vi "_builtins_arrange_panel.vi"(8 "error in (no error)":errorcluster, 10 "Arrange":T1, 11 "VI Refnum in":refnum<vi>) -> (0 "error out":errorcluster, 3 "VI Refnum out":refnum<vi>)   [LabVIEW 2019, in "Script.lvlib"]
doc: "Arranges the selected controls to the panel grid by left or top edges (hold shift). If nothing is selected, this will arrange all the controls on the panel into columns with a dead zone offset from the panel origin.\n\nCreated by: Ryan Pacini"
uses:
  Script.lvlib
  _builtins_arrange.ctl
  _builtins_align.ctl
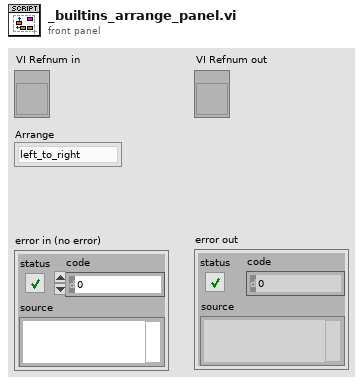
[diagram p1: front panel]
types:
  T1 = typedef "Script.lvlib/_builtins_arrange.ctl" = enum8{"left_to_right", "right_to_left"}
  T2 = typedef "Script.lvlib/_builtins_align.ctl" = enum8{"Top Edges", "Vertical Centers", "Bottom Edges", "Left Edges", "Horizontal Centers", "Right Edges"}
  T3 = typedef "LVRectTypeDef.ctl" = cluster{"Left":i16, "Top":i16, "Right":i16, "Bottom":i16}
  T4 = typedef "LVPositionTypeDef.ctl" = cluster{"Left":i32, "Top":i32}
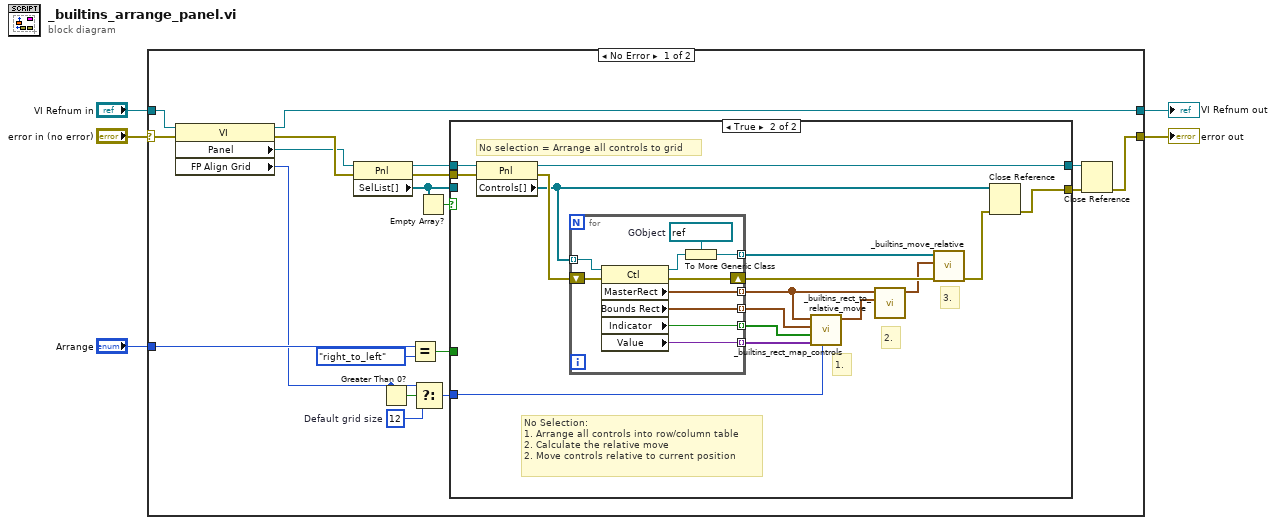
[diagram p0: block diagram]
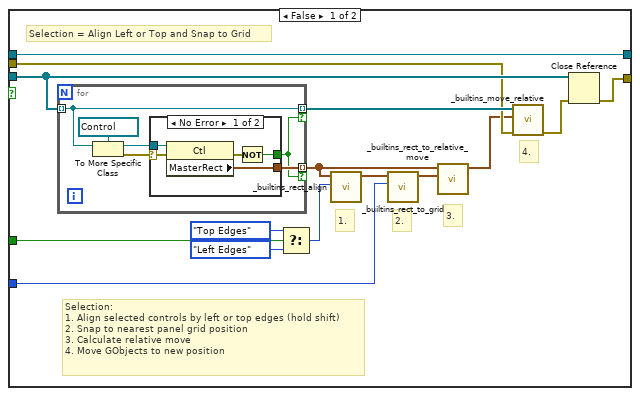
[diagram p2: hidden frame]
diagram:
  n1 = case shown="No Error" "error in (no error)" {
    selector: "error in (no error)" -> [w23 w77]
    tunnel: "VI Refnum in" -> [w24 w78]
    tunnel: [w18 w78] -> w4
    tunnel: [w19 w77] -> w2
    tunnel: "Arrange" -> [w11 _]
    frame No Error {
      w8 = 12  # Default grid size
      n2 = property class="VI"(reference=w24, error in=w23) -> (reference out=w18:refnum<vi>, error out=w22:errorcluster, "Panel"=w21:refnum<vi>, "FP Align Grid"=w7:i32)
      n3 = property class="Pnl"(reference=w21, error in=w22) -> (reference out=w13:refnum<vi>, error out=w16:errorcluster, "SelList[]"=w17:refnum<vi>[])
      n4 = Greater Than 0?(x=w7) -> (x > 0?=w9:bool)
      n5 = Equal?(x=w11, y=_builtins_arrange."right_to_left") -> (x = y?=w10:bool)
      n6 = Select(t=w7, s=w9, f=w8) -> (s? t:f=w6:i32)
      n7 = Empty Array?(array=w17) -> (empty?=w15:bool)
      n8 = case shown="True" w15 {
        tunnel: [w39 w58] -> w20
        tunnel: w17 -> [w36 _]
        tunnel: w16 -> [w32 w64]
        tunnel: [w31 w65] -> w14
        tunnel: w13 -> [w31 w66]
        tunnel: w6 -> [w28 w55]
        tunnel: w10 -> [w29 _]
        frame False {
          # "3."
          # "Selection:\n1. Align selected controls by left or top edges (hold shift)\n2. Snap to nearest panel grid position\n3. Calculate relative move\n4. Move GObjects to new position"
          # "2."
          # "4."
          # "1."
          # "Selection = Align Left or Top and Snap to Grid"
          n9 = for {
            tunnel: w36 -> [w40] mode=indexing
            tunnel: [w40] -> w38 mode=indexing if=w41
            tunnel: [w44] -> w27 mode=indexing if=w41
            n10 = To More Specific Class(target class=refnum<vi> refnum, reference=w40) -> (specific class reference=w42:refnum<vi>, error out=w43:errorcluster)  [unwired: 1 in]
            n11 = case shown="No Error" w43 {
              selector: w43 -> [w49 _]
              tunnel: [w50 _] -> w44
              tunnel: w42 -> [w48 _]
              tunnel: [w47 _] -> w41
              frame No Error {
                n12 = property class="Ctl"(reference=w48, error in=w49) -> (error out=w46:errorcluster, "MasterRect"=w50:T3)  [unwired: 1 out]
                n13 = Not(x=w46) -> (.not. x?=w47:bool)
              }
              frame Error {
              }
            }
          }
          n14 = Select(t=_builtins_align."Top Edges" ("Align Type"), s=w29, f=_builtins_align."Left Edges" ("Align Type")) -> (s? t:f=w33:T2)
          n15 = call "_builtins_rect_align.vi"("Align Type"=w33, "Rects in"=w27) -> ("Resolved Rects out"=w30:T3[])  [unwired: 9 in]
          n16 = call "_builtins_rect_to_grid.vi"("Grid Size (12px)"=w28, "Rects in"=w30) -> ("Resolved Rects out"=w26:T3[])  [unwired: 9 in]
          n17 = call "_builtins_rect_to_relative_move.vi"("End Rects out"=w26, "Start Rects in"=w27) -> ("Relative Move"=w25:T4[])  [unwired: 9 in]
          n18 = call "_builtins_move_relative.vi"("error in (no error)"=w32, "Relative Moves in"=w25, "GObjects in"=w38) -> ("error out"=w37:errorcluster)  [unwired: 7 in, 1 out]
          n19 = Close Reference(reference=w36, error in (no error)=w37) -> (error out=w39:errorcluster)
        }
        frame True {
          # "2."
          # "1."
          # "No Selection:\n1. Arrange all controls into row/column table\n2. Calculate the relative move\n2. Move controls relative to current position"
          # "3."
          # "No selection = Arrange all controls to grid"
          n20 = property class="Pnl"(reference=w66, error in=w64) -> (reference out=w65:refnum<vi>, error out=w63:errorcluster, "Controls[]"=w59:refnum<vi>[])
          n21 = for {
            shift-right: [w75] -> w61
            shift-left: w63 -> [w76]
            tunnel: w59 -> [w74] mode=indexing
            tunnel: [w73] -> w57 mode=indexing
            tunnel: [w72] -> w56 mode=indexing
            tunnel: [w70] -> w60 mode=indexing
            tunnel: [w68] -> w54 mode=indexing
            tunnel: [w67] -> w52 mode=indexing
            w69 = refnum<vi> refnum  # GObject
            n22 = property class="Ctl"(reference=w74, error in=w76) -> (reference out=w71:refnum<vi>, error out=w75:errorcluster, "MasterRect"=w68:T3, "Bounds Rect"=w73:T3, "Indicator"=w72:bool, "Value"=w67:variant)
            n23 = To More Generic Class(target class=w69, reference=w71) -> (generic class reference=w70:refnum<vi>)
          }
          n24 = call "_builtins_rect_map_controls.vi"("Grid Size (12px)"=w55, "Values"=w52, "Indicators"=w56, "TotalBndRects"=w57, "MasterBndRects in"=w54) -> ("Resolved MasterBndRects out"=w51:T3[])  [unwired: 6 in]
          n25 = call "_builtins_rect_to_relative_move.vi"("End Rects out"=w51, "Start Rects in"=w54) -> ("Relative Move"=w53:T4[])  [unwired: 9 in]
          n26 = call "_builtins_move_relative.vi"("error in (no error)"=w61, "Relative Moves in"=w53, "GObjects in"=w60) -> ("error out"=w62:errorcluster)  [unwired: 7 in, 1 out]
          n27 = Close Reference(reference=w59, error in (no error)=w62) -> (error out=w58:errorcluster)
        }
      }
      n28 = Close Reference(reference=w14, error in (no error)=w20) -> (error out=w19:errorcluster)
    }
    frame Error {
    }
  }
  "VI Refnum out" <- w4
  "error out" <- w2
